vi "Set Property.vi"(0 "Session Handle in":T1, 5 "resources":string, 7 "property":refnum<k21>, 9 "property value":bool, 11 "error in (no error)":errorcluster) -> (4 "Session Handle out":T1, 15 "error out":errorcluster)   [LabVIEW 2015, in "SLSC Switch.lvlib" / "SLSC Session.lvclass"]
uses:
  SLSC Session.lvclass
  Typedefs/Session Handle.ctl
  SLSC Session.lvclass/SLSC Session.ctl
  <vilib>/SLSC/Set Generic Property (Bool).vi
  <vilib>/SLSC/SLSC.lvlib
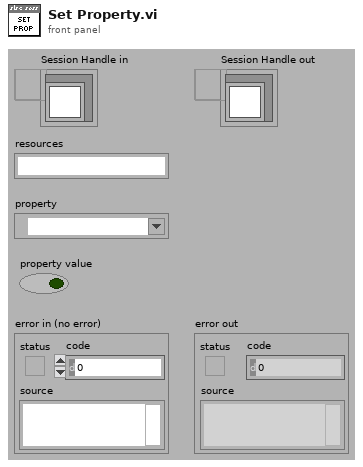
[diagram p1: front panel]
types:
  T1 = typedef "SLSC Switch.lvlib/SLSC Session.lvclass/Session Handle.ctl" = refnum<data-value>
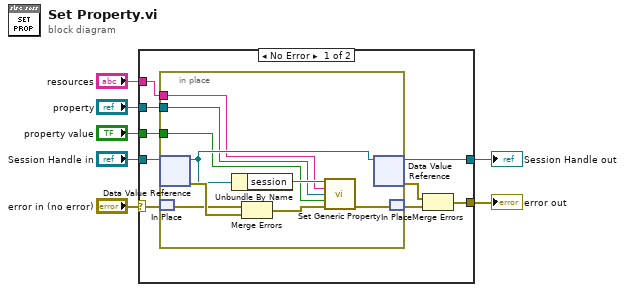
[diagram p0: block diagram]
diagram:
  n1 = case shown="No Error" "error in (no error)" {
    selector: "error in (no error)" -> [w11 w26]
    tunnel: "Session Handle in" -> [w16 w27]
    tunnel: [w15 w27] -> w6
    tunnel: [w12 w26] -> w5
    tunnel: "property value" -> [w10 _]
    tunnel: "resources" -> [w9 _]
    tunnel: "property" -> [w8 _]
    frame No Error {
      n2 = in-place {
        in-place-border: w10 -> [w19]
        in-place-border: w9 -> [w17]
        in-place-border: w8 -> [w18]
        n3 = in-place-dvr #1(w16) -> (w23:refnum<class "SLSC Session.lvclass">, w25:errorcluster)
        n4 = in-place-match #2(w11) -> (w24:errorcluster)
        n5 = Unbundle By Name(w23) -> ("session"=w22:refnum<k21>)
        n6 = Merge Errors(w24, w25) -> (w21:errorcluster)
        n7 = call-poly <vilib>:"Set Generic Property.vi"("session in"=w22, "resources"=w17, "property"=w18, "property value"=w19, "error in (no error)"=w21) -> ("error out"=w20:errorcluster)  [unwired: 9 in, 1 out]
        n8 = in-place-dvr #1(w23) -> (w15:T1, w13:errorcluster)
        n9 = in-place-match #2(w20) -> (w14:errorcluster)
      }
      n10 = Merge Errors(w13, w14) -> (w12:errorcluster)
    }
    frame Error {
    }
  }
  "Session Handle out" <- w6
  "error out" <- w5
